vi "Test C.vi"(8 "error in (no error)":errorcluster) -> (0 "error out":errorcluster)   [LabVIEW 2019, in "Simple Example(Station2).lvlib"]
uses:
  b65cedc0-6f88-47fe-863c-f92be18f8f6a.vi
  941f3686-130e-45b0-8e30-bc4649ace6bb.vi
  LVUT Global 1.vi
  <vilib>/Utility/Data Type/Get Type Information.vi
  <vilib>/Utility/error.llb/Trim Whitespace.vi
  Equal Value.vi
  Simple Example(Station2).lvlib
  Unit Test Engine Tools.lvlib
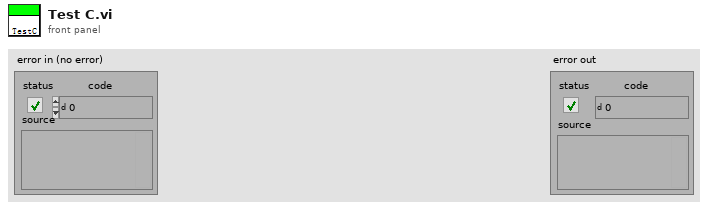
[diagram p1: front panel]
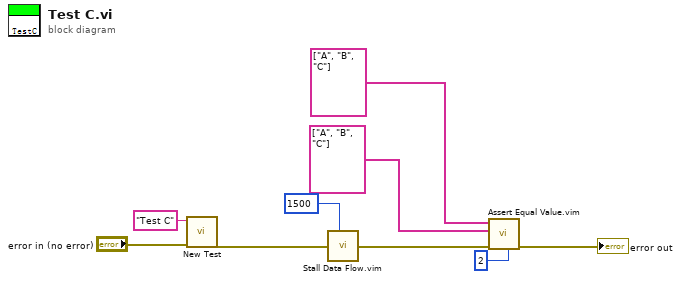
[diagram p0: block diagram]
diagram:
  n1 = call "New Test.vi"("error in (no error)"="error in (no error)", "Test"="Test C") -> ("error out"=w7:errorcluster)  [unwired: 9 in]
  n2 = call "Stall Data Flow.vim"("value in"=w7, "milliseconds to wait"=u32 1500) -> ("value out"=w4:errorcluster)  [unwired: 1 out]
  n3 = call "Assert Equal Value.vim"("precision (2)"=i16 2 ("precision (6)"), "error in (no error)"=w4, "Y"=string[] ["A", "B", "C"], "X"=string[] ["A", "B", "C"]) -> ("error out"=→"error out":errorcluster)  [unwired: 7 in]
